vi "FileNameIso8601.vi"(10 "Extension (.log)":string=".log", 11 "Prefix ('')":string) -> (3 "FileName":string)   [LabVIEW 2022 SP3, in "DateTime.lvlib"]
uses:
  DateTime.lvlib
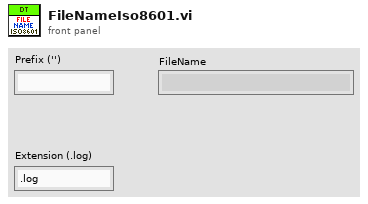
[diagram p1: front panel]
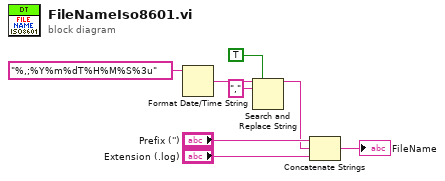
[diagram p0: block diagram]
diagram:
  n1 = Format Date/Time String(time format string (%c)="%,;%Y%m%dT%H%M%S%3u") -> (date/time string=w7:string)  [unwired: 2 in]
  n2 = Search and Replace String(replace all?=TRUE ("replace all? (F)"), input string=w7, search string=",") -> (result string=w2:string)  [unwired: 5 in, 3 out]
  n3 = Concatenate Strings("Prefix ('')", w2, "Extension (.log)") -> (→"FileName":string)
